vi "Scale Arbitrary Waveform.vi"(8 "error in (no error)":errorcluster, 10 "Arbitrary Waveform Data":dbl[](array[numeric]), 11 "VISA resource name":refnum<visa-resource-name>) -> (0 "error out":errorcluster, 2 "Scaled Arbitrary Waveform Data":i16[](array[numeric]), 3 "VISA resource name out":refnum<visa-resource-name>)   [LabVIEW 2012, in "Agilent 33XXX Series.lvlib"]
doc: "This VI scales a data array so that the maximum (positive or negative) value in the array corresponds to the maximum allowed value (positive or negative) for the instrument.\n\n33120a: -2047 to 2047\n33220a/33250a: -8191 to 8191"
uses:
  Agilent 33XXX Series.lvlib
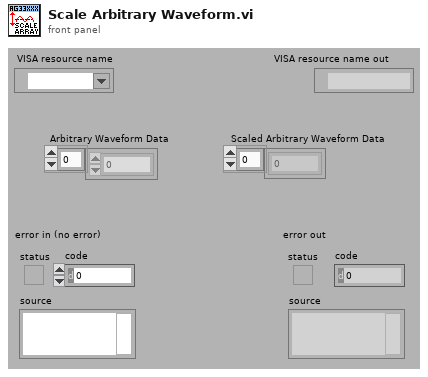
[diagram p1: front panel]
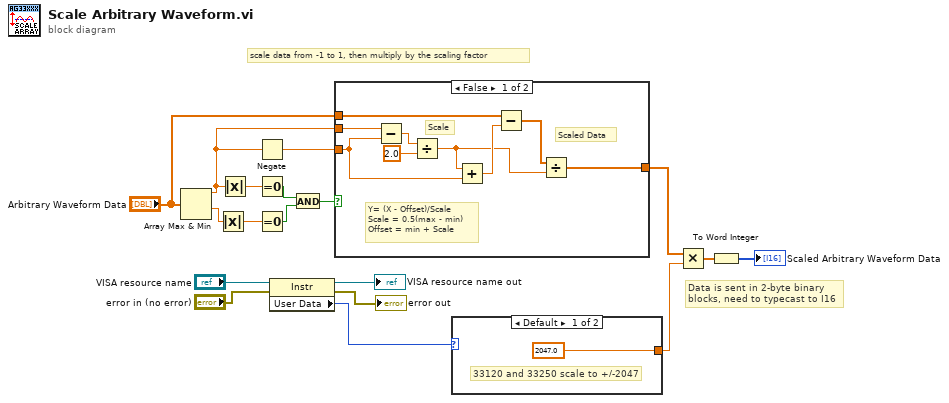
[diagram p0: block diagram]
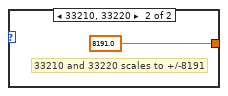
[diagram p2: hidden frame]
diagram:
  # "Data is sent in 2-byte binary blocks, need to typecast to I16"
  # "scale data from -1 to 1, then multiply by the scaling factor"
  n1 = Array Max & Min(array="Arbitrary Waveform Data") -> (max value=w2:dbl, min value=w11:dbl)  [unwired: 2 out]
  n2 = Absolute Value(x=w11) -> (abs(x)=w14:dbl)
  n3 = Absolute Value(x=w2) -> (abs(x)=w13:dbl)
  n4 = Negate(x=w2) -> (-x=w1:dbl)
  n5 = Equal To 0?(x=w13) -> (x = 0?=w16:bool)
  n6 = Equal To 0?(x=w14) -> (x = 0?=w15:bool)
  n7 = property class="Instr"(reference="VISA resource name", error in="error in (no error)") -> (reference out=→"VISA resource name out":refnum<visa-resource-name>, error out=→"error out":errorcluster, "User Data"=w4:u32)
  n8 = And(x=w16, y=w15) -> (x .and. y?=w12:bool)
  n9 = case shown="False" w12 {
    tunnel: w2 -> [w27 _]
    tunnel: "Arbitrary Waveform Data" -> [w24 w28]
    tunnel: [w20 w28] -> w9
    tunnel: w1 -> [w19 _]
    frame False {
      # "Y= (X - Offset)/Scale\nScale = 0.5(max - min)\nOffset = min + Scale"
      # "Scale"
      # "Scaled Data"
      n10 = Subtract(x=w27, y=w19) -> (x-y=w26:dbl)
      n11 = Divide(x=w26, y=2.0) -> (x/y=w21:dbl)
      n12 = Add(x=w21, y=w19) -> (x+y=w23:dbl)
      n13 = Subtract(x=w24, y=w23) -> (x-y=w22:dbl[])
      n14 = Divide(x=w22, y=w21) -> (x/y=w20:dbl[])
    }
    frame True {
      # "This case occurs when all the data in the table\nare zeros, thus, the maximum and the minimum\nare the same and no division required."
    }
  }
  n15 = case shown="Default" w4 {
    tunnel: [2047.0 ("y") 8191.0 ("y")] -> w3
    frame Default {
      # "33120 and 33250 scale to +/-2047"
    }
    frame 33210, 33220 {
      # "33210 and 33220 scales to +/-8191"
    }
  }
  n16 = Multiply(x=w9, y=w3) -> (x*y=w17:dbl[])
  n17 = To Word Integer(number=w17) -> (16bit integer=→"Scaled Arbitrary Waveform Data":i16[])
